vi "Create Class Items.vi"(7 "Template Class Items":refnum<vi>[](array[refnum]), 8 "error in (no error)":errorcluster, 11 "QControl Creation in":refnum<class "QControl Creation.lvclass">) -> (0 "error out":errorcluster, 3 "QControl Creation out":refnum<class "QControl Creation.lvclass">)   [LabVIEW 2015, in "QControl Creation.lvclass"]
doc: "<b> </b> <b> </b>\n©2016 Q Software Innovations, LLC (QSI)\nwritten by Quentin Alldredge\nproduced in LabVIEW 2015\n\nsupport@qsoftwareinnovations.com\nwww.qsoftwareinnovations.com\n\nAll rights reserved.\n\nRedistribution and use in source and binary forms, with or without modification, are permitted provided that the following conditions are met:\n\n * Redistributions of source code must retain the above copyright notice, this list of conditions and the following disclaimer.\n * Redistributions in binary form must reproduce the above copyright notice, this list of conditions and the following disclaimer in the documentation and/or other materials provided with the distribution.\n * Neither the name of Q Software Innovations, LLC. nor the names of its contributors may be used to endorse or promote products derived from this software without specific prior written permission.\n\nTHIS SOFTWARE IS PROVIDED BY THE COPYRIGHT HOLDERS AND CONTRIBUTORS \"AS IS\" AND ANY EXPRESS OR IMPLIED WARRANTIES, INCLUDING, BUT NOT LIMITED TO, THE IMPLIED WARRANTIES OF MERCHANTABILITY AND FITNESS FOR A PARTICULAR PURPOSE ARE DISCLAIMED. IN NO EVENT SHALL THE COPYRIGHT OWNER OR CONTRIBUTORS BE LIABLE FOR ANY DIRECT, INDIRECT, INCIDENTAL, SPECIAL, EXEMPLARY, OR CONSEQUENTIAL DAMAGES (INCLUDING, BUT NOT LIMITED TO, PROCUREMENT OF SUBSTITUTE GOODS OR SERVICES; LOSS OF USE, DATA, OR PROFITS; OR BUSINESS INTERRUPTION) HOWEVER CAUSED AND ON ANY THEORY OF LIABILITY, WHETHER IN CONTRACT, STRICT LIABILITY, OR TORT (INCLUDING NEGLIGENCE OR OTHERWISE) ARISING IN ANY WAY OUT OF THE USE OF THIS SOFTWARE, EVEN IF ADVISED OF THE POSSIBILITY OF SUCH DAMAGE."
uses:
  QControl Creation.lvclass
  <vilib>/ErrorRing/Error Ring.xnode
  New QControl Info/New QControl Info.lvclass
  <vilib>/Utility/error.llb/Error Cluster From Error Code.vi
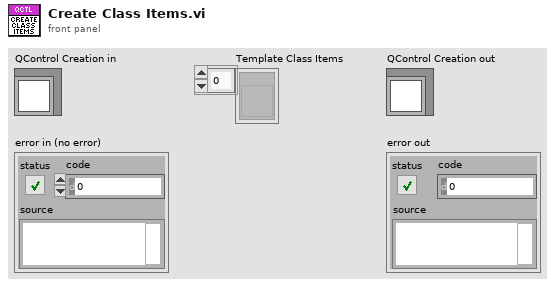
[diagram p1: front panel]
types:
  T1 = enum32{"invalid VI type", "Standard VI", "Control VI", "Global VI", "Polymorphic VI", "Configuration VI", "SubSystem", "Facade VI", "Method VI", "Statechart Diagram VI"}
  T2 = enum32{"invalid scope", "public", "private", "protected", "community"}
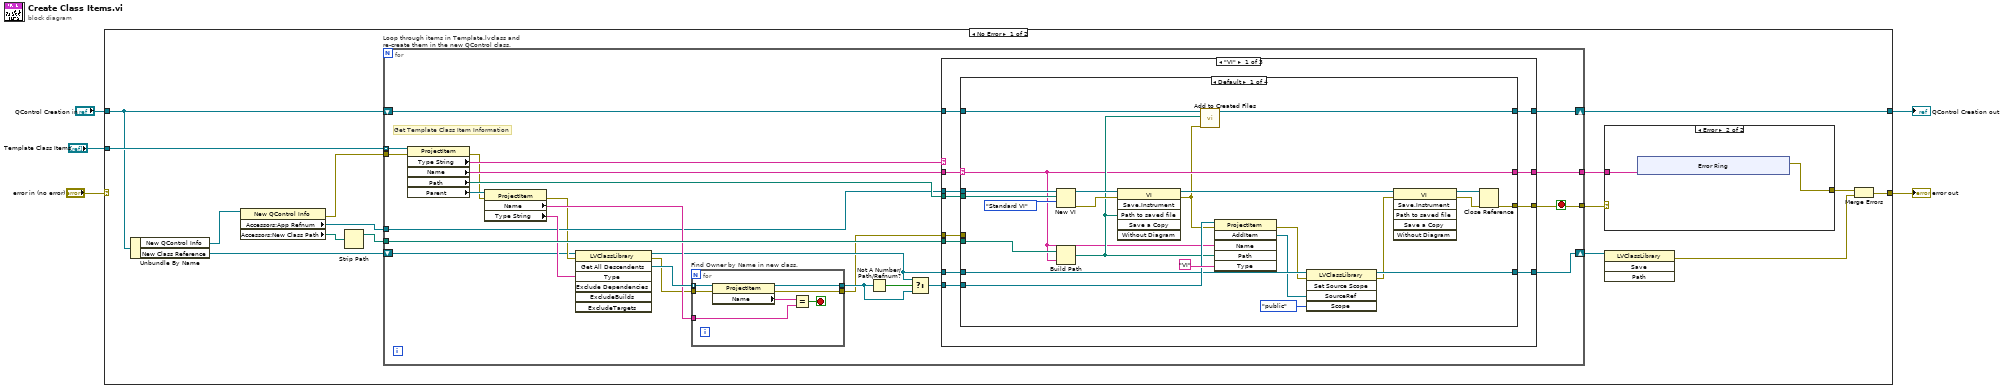
[diagram p0: block diagram]
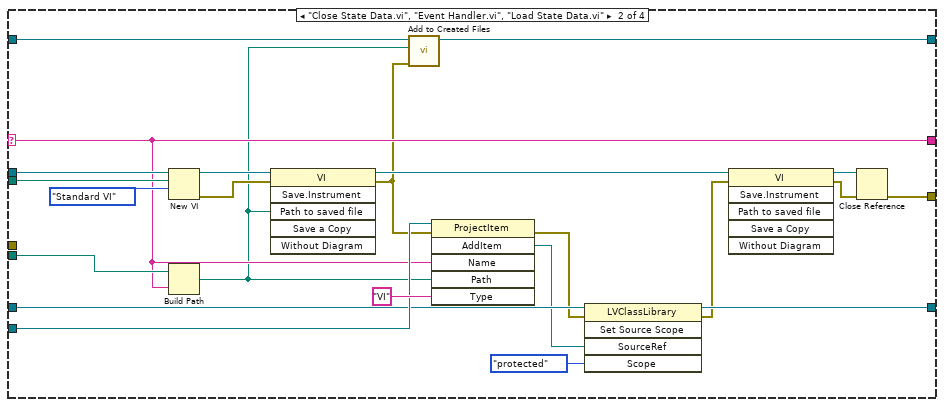
[diagram p3: hidden frame]
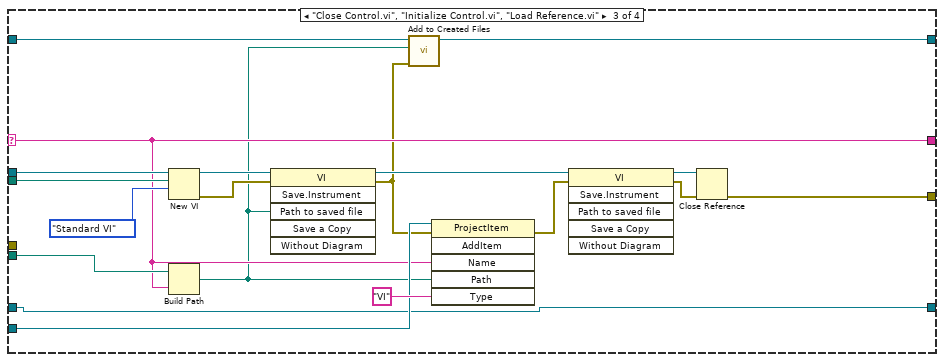
[diagram p4: hidden frame]
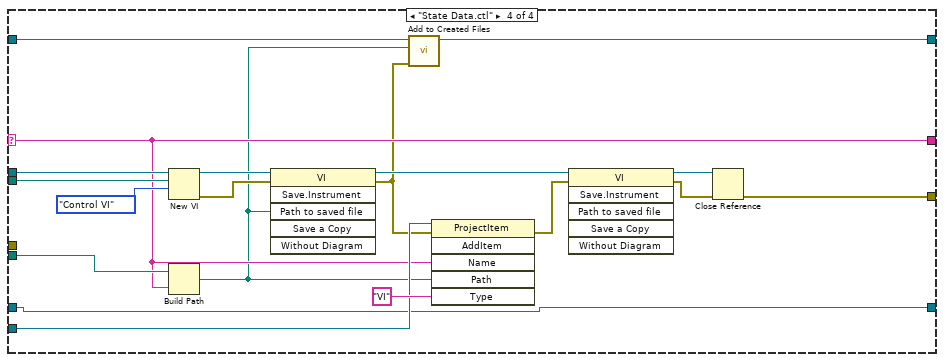
[diagram p5: hidden frame]
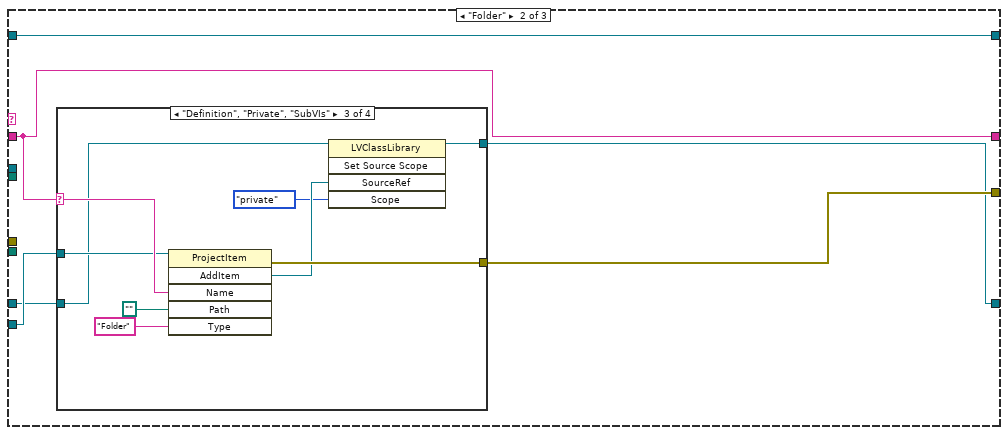
[diagram p6: hidden frame]
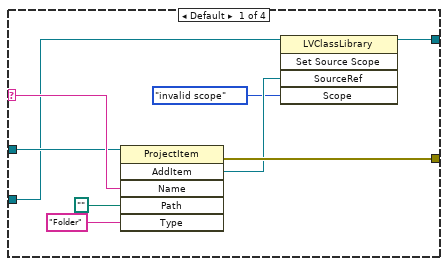
[diagram p7: hidden frame]
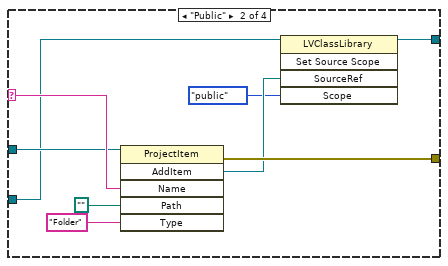
[diagram p8: hidden frame]
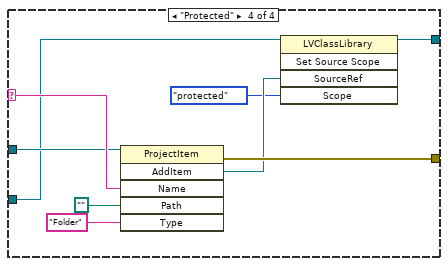
[diagram p9: hidden frame]
diagram:
  n1 = case shown="No Error" "error in (no error)" {
    selector: "error in (no error)" -> [_ w205]
    tunnel: "Template Class Items" -> [w20 _]
    tunnel: [w18 w205] -> w4
    tunnel: "QControl Creation in" -> [w11 w204]
    tunnel: [w10 w204] -> w1
    frame No Error {
      n2 = Unbundle By Name(w11) -> ("New QControl Info"=w9:refnum<data-value>, "New Class Reference"=w12:refnum<vi>)
      n3 = property class="New QControl Info"(reference=w9) -> (error out=w6:errorcluster, "Accessors:App Refnum"=w8:refnum<vi>, "Accessors:New Class Path"=w7:path)  [unwired: 1 in, 1 out]
      n4 = Strip Path(path=w7) -> (stripped path=w13:path)  [unwired: 1 out]
      n5 = for "Loop through items in Template.lvclass and re-create them in the new QControl class." {
        tunnel: w20 -> [w55] mode=indexing
        tunnel: w13 -> [w52]
        shift-right: [w42] -> w17
        shift-left: w12 -> [w37]
        tunnel: w8 -> [w41]
        tunnel: [w36] -> w15
        tunnel: [w35] -> w19
        shift-right: [w33] -> w10
        shift-left: w11 -> [w32]
        tunnel: w6 -> [w31]
        stop <- w36 stop-if-true
        # "Get Template Class Item Information"
        n6 = property class="ProjectItem"(reference=w55, error in=w31) -> (error out=w40:errorcluster, "Type String"=w54:string, "Name"=w50:string, "Path"=w53:path, "Parent"=w49:refnum<vi>)  [unwired: 1 out]
        n7 = property class="ProjectItem"(reference=w49, error in=w40) -> (error out=w39:errorcluster, "Name"=w48:string, "Type String"=w47:string)  [unwired: 1 out]
        n8 = invoke class="LVClassLibrary" method="Get All Descendents"(reference=w37, error in=w39, "Type"=w47) -> (reference out=w43:refnum<vi>, error out=w38:errorcluster, "All Descendents"=w51:refnum<vi>[])  [unwired: 4 in, 4 out]
        n9 = for "Find Owner by Name in new class." {
          tunnel: w51 -> [w62] mode=indexing
          tunnel: w48 -> [w60]
          tunnel: [w59] -> w44
          tunnel: w38 -> [w57]
          tunnel: [w56] -> w34
          stop <- w58 stop-if-true
          n10 = property class="ProjectItem"(reference=w62, error in=w57) -> (reference out=w59:refnum<vi>, error out=w56:errorcluster, "Name"=w61:string)
          n11 = Equal?(x=w61, y=w60) -> (x = y?=w58:bool)
        }
        n12 = Not A Number/Path/Refnum?(number/path/refnum=w44) -> (NaN/Path/Refnum?=w46:bool)
        n13 = Select(t=w43, s=w46, f=w44) -> (s? t:f=w45:refnum<vi>)
        n14 = case shown="\"VI\"" w54 {
          tunnel: w50 -> [w67 w160 w202]
          tunnel: w53 -> [w74 _ _]
          tunnel: w52 -> [w73 _ _]
          tunnel: w45 -> [w72 w163 _]
          tunnel: [w69 w164 _] -> w36
          tunnel: w43 -> [w71 w162 w203]
          tunnel: [w70 w161 w203] -> w42
          tunnel: w41 -> [w68 _ _]
          tunnel: [w65 w160 w202] -> w35
          tunnel: w34 -> [w66 _ _]
          tunnel: [w64 w159 w201] -> w33
          tunnel: w32 -> [w63 w159 w201]
          frame "VI" {
            n15 = case shown="Default" w67 {
              selector: w67 -> [w77 w103 w125 w144]
              tunnel: w74 -> [w96 w119 w138 w157]
              tunnel: w73 -> [w94 w117 w136 w155]
              tunnel: w72 -> [w93 w116 w135 w154]
              tunnel: w71 -> [w92 w115 w134 w153]
              tunnel: [w90 w113 w134 w153] -> w70
              tunnel: [w78 w102 w130 w150] -> w69
              tunnel: w68 -> [w86 w109 w129 w149]
              tunnel: w66 -> [_ _ _ _]
              tunnel: [w77 w103 w125 w144] -> w65
              tunnel: [w79 w101 w122 w140] -> w64
              tunnel: w63 -> [w76 w100 w123 w143]
              frame Default {
                n16 = New VI(9:T1."Standard VI" ("vi type (standard vi)"), 10:w96, 11:w86) -> (0:w85:errorcluster, 3:w97:refnum<vi>)  [unwired: 4 in]
                n17 = Build Path(base path=w94, name or relative path=w77) -> (appended path=w80:path)
                n18 = invoke class="VI" method="Save.Instrument"(reference=w97, error in=w85, "Path to saved file"=w80) -> (reference out=w89:refnum<vi>, error out=w75:errorcluster)  [unwired: 3 in, 4 out]
                n19 = call "Add to Created Files.vi"("error in (no error)"=w75, "Path to Add"=w80, "QControl Creation in"=w76) -> ("QControl Creation out"=w79:refnum<class "QControl Creation.lvclass">)  [unwired: 8 in]
                n20 = invoke class="ProjectItem" method="AddItem"(reference=w93, error in=w75, "Name"=w77, "Path"=w80, "Type"="VI") -> (error out=w84:errorcluster, "AddItem"=w91:refnum<vi>)  [unwired: 1 in, 4 out]
                n21 = invoke class="LVClassLibrary" method="Set Source Scope"(reference=w92, error in=w84, "SourceRef"=w91, "Scope"=T2."public" ("scope")) -> (reference out=w90:refnum<vi>, error out=w83:errorcluster)  [unwired: 1 in, 3 out]
                n22 = invoke class="VI" method="Save.Instrument"(reference=w89, error in=w83) -> (reference out=w88:refnum<vi>, error out=w87:errorcluster)  [unwired: 4 in, 4 out]
                n23 = Close Reference(reference=w88, error in (no error)=w87) -> (error out=w78:errorcluster)
              }
              frame "Close State Data.vi", "Event Handler.vi", "Load State Data.vi" {
                n24 = New VI(9:T1."Standard VI" ("vi type (standard vi)"), 10:w119, 11:w109) -> (0:w108:errorcluster, 3:w120:refnum<vi>)  [unwired: 4 in]
                n25 = Build Path(base path=w117, name or relative path=w103) -> (appended path=w99:path)
                n26 = invoke class="VI" method="Save.Instrument"(reference=w120, error in=w108, "Path to saved file"=w99) -> (reference out=w112:refnum<vi>, error out=w98:errorcluster)  [unwired: 3 in, 4 out]
                n27 = call "Add to Created Files.vi"("error in (no error)"=w98, "Path to Add"=w99, "QControl Creation in"=w100) -> ("QControl Creation out"=w101:refnum<class "QControl Creation.lvclass">)  [unwired: 8 in]
                n28 = invoke class="ProjectItem" method="AddItem"(reference=w116, error in=w98, "Name"=w103, "Path"=w99, "Type"="VI") -> (error out=w107:errorcluster, "AddItem"=w114:refnum<vi>)  [unwired: 1 in, 4 out]
                n29 = invoke class="LVClassLibrary" method="Set Source Scope"(reference=w115, error in=w107, "SourceRef"=w114, "Scope"=T2."protected" ("scope")) -> (reference out=w113:refnum<vi>, error out=w106:errorcluster)  [unwired: 1 in, 3 out]
                n30 = invoke class="VI" method="Save.Instrument"(reference=w112, error in=w106) -> (reference out=w111:refnum<vi>, error out=w110:errorcluster)  [unwired: 4 in, 4 out]
                n31 = Close Reference(reference=w111, error in (no error)=w110) -> (error out=w102:errorcluster)
              }
              frame "Close Control.vi", "Initialize Control.vi", "Load Reference.vi" {
                n32 = New VI(9:T1."Standard VI" ("vi type (standard vi)"), 10:w138, 11:w129) -> (0:w128:errorcluster, 3:w139:refnum<vi>)  [unwired: 4 in]
                n33 = Build Path(base path=w136, name or relative path=w125) -> (appended path=w121:path)
                n34 = invoke class="VI" method="Save.Instrument"(reference=w139, error in=w128, "Path to saved file"=w121) -> (reference out=w133:refnum<vi>, error out=w124:errorcluster)  [unwired: 3 in, 4 out]
                n35 = call "Add to Created Files.vi"("error in (no error)"=w124, "Path to Add"=w121, "QControl Creation in"=w123) -> ("QControl Creation out"=w122:refnum<class "QControl Creation.lvclass">)  [unwired: 8 in]
                n36 = invoke class="ProjectItem" method="AddItem"(reference=w135, error in=w124, "Name"=w125, "Path"=w121, "Type"="VI") -> (error out=w127:errorcluster)  [unwired: 1 in, 5 out]
                n37 = invoke class="VI" method="Save.Instrument"(reference=w133, error in=w127) -> (reference out=w132:refnum<vi>, error out=w131:errorcluster)  [unwired: 4 in, 4 out]
                n38 = Close Reference(reference=w132, error in (no error)=w131) -> (error out=w130:errorcluster)
              }
              frame "State Data.ctl" {
                n39 = New VI(9:T1."Control VI" ("vi type (standard vi)"), 10:w157, 11:w149) -> (0:w148:errorcluster, 3:w158:refnum<vi>)  [unwired: 4 in]
                n40 = Build Path(base path=w155, name or relative path=w144) -> (appended path=w141:path)
                n41 = invoke class="VI" method="Save.Instrument"(reference=w158, error in=w148, "Path to saved file"=w141) -> (reference out=w145:refnum<vi>, error out=w142:errorcluster)  [unwired: 3 in, 4 out]
                n42 = call "Add to Created Files.vi"("error in (no error)"=w142, "Path to Add"=w141, "QControl Creation in"=w143) -> ("QControl Creation out"=w140:refnum<class "QControl Creation.lvclass">)  [unwired: 8 in]
                n43 = invoke class="ProjectItem" method="AddItem"(reference=w154, error in=w142, "Name"=w144, "Path"=w141, "Type"="VI") -> (error out=w146:errorcluster)  [unwired: 1 in, 5 out]
                n44 = invoke class="VI" method="Save.Instrument"(reference=w145, error in=w146) -> (reference out=w152:refnum<vi>, error out=w151:errorcluster)  [unwired: 4 in, 4 out]
                n45 = Close Reference(reference=w152, error in (no error)=w151) -> (error out=w150:errorcluster)
              }
            }
          }
          frame "Folder" {
            n46 = case shown="\"Definition\", \"Private\", \"SubVIs\"" w160 {
              selector: w160 -> [w173 w182 w191 w200]
              tunnel: [w170 w179 w188 w197] -> w164
              tunnel: w163 -> [w169 w178 w187 w196]
              tunnel: w162 -> [w168 w177 w186 w195]
              tunnel: [w166 w175 w184 w193] -> w161
              frame Default {
                n47 = invoke class="ProjectItem" method="AddItem"(reference=w169, "Name"=w173, "Path"=path "", "Type"="Folder") -> (error out=w170:errorcluster, "AddItem"=w167:refnum<vi>)  [unwired: 2 in, 4 out]
                n48 = invoke class="LVClassLibrary" method="Set Source Scope"(reference=w168, "SourceRef"=w167, "Scope"=T2."invalid scope" ("scope")) -> (reference out=w166:refnum<vi>)  [unwired: 2 in, 4 out]
              }
              frame "Public" {
                n49 = invoke class="ProjectItem" method="AddItem"(reference=w178, "Name"=w182, "Path"=path "", "Type"="Folder") -> (error out=w179:errorcluster, "AddItem"=w176:refnum<vi>)  [unwired: 2 in, 4 out]
                n50 = invoke class="LVClassLibrary" method="Set Source Scope"(reference=w177, "SourceRef"=w176, "Scope"=T2."public" ("scope")) -> (reference out=w175:refnum<vi>)  [unwired: 2 in, 4 out]
              }
              frame "Definition", "Private", "SubVIs" {
                n51 = invoke class="ProjectItem" method="AddItem"(reference=w187, "Name"=w191, "Path"=path "", "Type"="Folder") -> (error out=w188:errorcluster, "AddItem"=w185:refnum<vi>)  [unwired: 2 in, 4 out]
                n52 = invoke class="LVClassLibrary" method="Set Source Scope"(reference=w186, "SourceRef"=w185, "Scope"=T2."private" ("scope")) -> (reference out=w184:refnum<vi>)  [unwired: 2 in, 4 out]
              }
              frame "Protected" {
                n53 = invoke class="ProjectItem" method="AddItem"(reference=w196, "Name"=w200, "Path"=path "", "Type"="Folder") -> (error out=w197:errorcluster, "AddItem"=w194:refnum<vi>)  [unwired: 2 in, 4 out]
                n54 = invoke class="LVClassLibrary" method="Set Source Scope"(reference=w195, "SourceRef"=w194, "Scope"=T2."protected" ("scope")) -> (reference out=w193:refnum<vi>)  [unwired: 2 in, 4 out]
              }
            }
          }
          frame Default {
          }
        }
      }
      n55 = case shown="Error" w15 {
        selector: w15 -> [w21 _]
        tunnel: w19 -> [_ w23]
        tunnel: [w21 w22] -> w14
        frame No Error {
        }
        frame Error {
          n56 = xnode "Error Ring"("parameter 0"=w23) -> ("error out"=w22:errorcluster)
        }
      }
      n57 = invoke class="LVClassLibrary" method="Save"(reference=w17) -> (error out=w16:errorcluster)  [unwired: 3 in, 3 out]
      n58 = Merge Errors(w14, w16) -> (w18:errorcluster)
    }
    frame Error {
    }
  }
  "error out" <- w4
  "QControl Creation out" <- w1
